vi "AO_init.vi"(0 "AOParameters":string[](array[string]), 1 "N_param":i32, 2 "N_moduls":i32, 5 "Parameters def":dbl[][](array[numeric]), 7 "Names def":string[][](array[string]), 9 "KFM":string[](array[string]), 12 "conninfo":T1={"host"="localhost", "port"="5432", "client_encoding"="WIN1251", "dbname"="data", "user"="postgres", "password"=""}, 13 "AOParamTable":string="fao_3") -> (4 "AO out":T2, 15 "error":errorcluster)   [LabVIEW 2019, in "Inputs.lvlib"]
uses:
  Inputs.lvlib
  Ctl/AO.ctl
  Ctl/Parameter State.ctl
  Database/ctl/Coninfo.ctl
  Database/PostgreSQL.lvlib
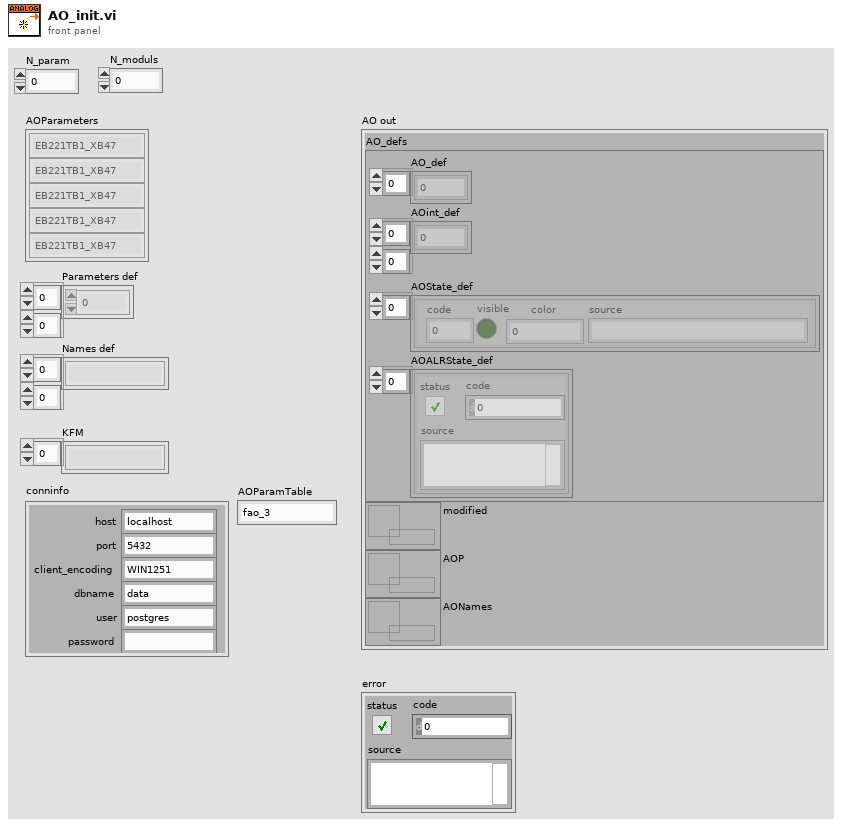
[diagram p1: front panel]
types:
  T1 = typedef "PostgreSQL.lvlib/Coninfo.ctl" = cluster{"host":string, "port":string, "client_encoding":string, "dbname":string, "user":string, "password":string}
  T2 = typedef "Inputs.lvlib/AO.ctl" = cluster{"AO_defs":cluster{"AO_def":dbl[], "AOint_def":u16[][], "AOState_def":T3[], "AOALRState_def":errorcluster[]}, "modified":refnum<data-value>, "AOP":refnum<data-value>, "AONames":refnum<data-value>}
  T3 = typedef "Inputs.lvlib/Parameter State.ctl" = cluster{"code":i32, "visible":bool, "color":u32, "source":string}
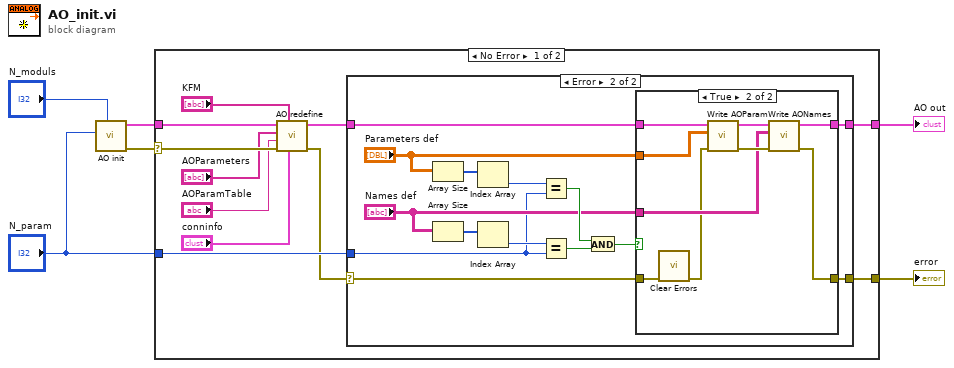
[diagram p0: block diagram]
diagram:
  n1 = call "AO init.vi"("N_moduls"="N_moduls", "N_param"="N_param") -> ("error"=w3:errorcluster, "AO"=w4:T2)  [unwired: 8 in]
  n2 = case shown="No Error" w3 {
    selector: w3 -> [w14 w46]
    tunnel: "N_param" -> [w16 _]
    tunnel: [w17 w46] -> w6
    tunnel: w4 -> [w13 w45]
    tunnel: [w15 w45] -> w2
    frame No Error {
      n3 = call "AO redefine.vi"("conninfo"="conninfo", "KFM"="KFM", "error in (no error)"=w14, "AOParamTable"="AOParamTable", "AOParameters"="AOParameters", "AO in"=w13) -> ("error"=w11:errorcluster, "AO out"=w12:T2)  [unwired: 4 in]
      n4 = case shown="Error" w11 {
        selector: w11 -> [w19 w24]
        tunnel: [w19 w25] -> w17
        tunnel: w16 -> [_ w26]
        tunnel: w12 -> [w18 w21]
        tunnel: [w18 w20] -> w15
        frame No Error {
        }
        frame Error {
          n5 = Array Size(array="Parameters def") -> (size(s)=w28:i32[])
          n6 = Array Size(array="Names def") -> (size(s)=w29:i32[])
          n7 = Index Array(array=w28) -> (element=w30:i32)  [unwired: 1 in]
          n8 = Index Array(array=w29) -> (element=w31:i32)  [unwired: 1 in]
          n9 = Equal?(x=w30, y=w26) -> (x = y?=w32:bool)
          n10 = Equal?(x=w31, y=w26) -> (x = y?=w33:bool)
          n11 = And(x=w32, y=w33) -> (x .and. y?=w22:bool)
          n12 = case shown="True" w22 {
            tunnel: "Parameters def" -> [_ w37]
            tunnel: "Names def" -> [_ w38]
            tunnel: [w34 w41] -> w25
            tunnel: w24 -> [w34 w39]
            tunnel: w21 -> [w35 w42]
            tunnel: [w35 w40] -> w20
            frame False {
            }
            frame True {
              n13 = call <vilib>:"Clear Errors.vi"("error in (no error)"=w39) -> ("error out"=w36:errorcluster)  [unwired: 5 in, 1 out]
              n14 = call "Write AOParam.vi"("error in (no error)"=w36, "AOParam"=w37, "AO in"=w42) -> ("error out"=w43:errorcluster, "AO out"=w44:T2)  [unwired: 7 in]
              n15 = call "Write AONames.vi"("error in (no error)"=w43, "AONames"=w38, "AO in"=w44) -> ("error out"=w41:errorcluster, "AO out"=w40:T2)  [unwired: 7 in]
            }
          }
        }
      }
    }
    frame Error {
    }
  }
  "AO out" <- w2
  "error" <- w6
